vi "Parse SSH_FXP_NAME.vi"(8 "error in":errorcluster, 11 "payload":u8[](array[numeric])) -> (0 "error out":errorcluster, 3 "files":T1[](array[typedef]) {"file attributes"."permissions" format="%04o"})   [LabVIEW 2020, in "NI_SFTP.lvlib"]
uses:
  <vilib>/net/SFTP/NI_SFTP.lvlib
  <vilib>/net/SFTP/API/Support/Name.ctl
  <vilib>/net/SFTP/API/Support/File Attributes.ctl
  f023bfa8-f8fb-3feb-c0fc-b0554016e43f.vi
  fe9cab8e-2cf0-3fe7-1c9b-f8983c6ade3f.vi
  248d59e0-ee9f-3fd5-30f8-f80d1baee43f.vi
  <vilib>/Bit Manipulation/Network-Order Bytes To Words Poly.vi
  <vilib>/Bit Manipulation/wrappers/Network-Order Bytes To Words/Network-Order Bytes To Words U32.vi
  <vilib>/net/SFTP/Low Level Connection/Low Level Connection.lvclass
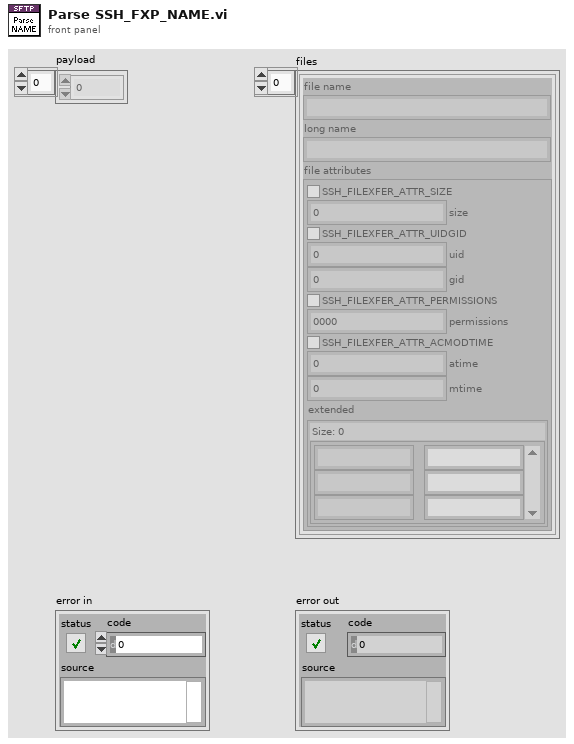
[diagram p1: front panel]
types:
  T1 = typedef "NI_SFTP.lvlib/Name.ctl" = cluster{"file name":string, "long name":string, "file attributes":T2}
  T2 = typedef "NI_SFTP.lvlib/File Attributes.ctl" = cluster{"SSH_FILEXFER_ATTR_SIZE":bool, "size":u64, "SSH_FILEXFER_ATTR_UIDGID":bool, "uid":u32, "gid":u32, "SSH_FILEXFER_ATTR_PERMISSIONS":bool, "permissions":u32, "SSH_FILEXFER_ATTR_ACMODTIME":bool, "atime":u32, "mtime":u32, "extended":map{string, string}}
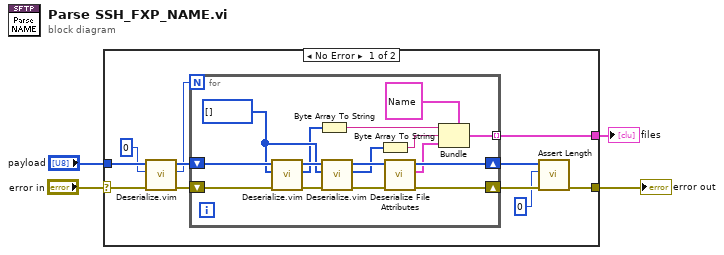
[diagram p0: block diagram]
diagram:
  n1 = case shown="No Error" "error in" {
    selector: "error in" -> [w14 w32]
    tunnel: [w8 w32] -> w3
    tunnel: "payload" -> [w15 _]
    tunnel: [w5 _] -> w1
    frame No Error {
      n2 = call "Deserialize.vim"("error in"=w14, "type"=u32 0, "bytes"=w15) -> ("error out"=w12:errorcluster, "value"=w6:u32, "remaining bytes"=w13:u8[])  [unwired: 6 in]
      n3 = for {
        N: w6 -> [_]
        shift-right: [w24] -> w9
        shift-left: w12 -> [w30]
        shift-right: [w25] -> w10
        shift-left: w13 -> [w31]
        tunnel: [w22] -> w5 mode=indexing
        w20 = u8[] [] ("payload")
        n4 = call "Deserialize.vim"("error in"=w30, "type"=w20, "bytes"=w31) -> ("error out"=w28:errorcluster, "value"=w19:u8[], "remaining bytes"=w29:u8[])  [unwired: 6 in]
        n5 = Byte Array To String(unsigned byte array=w19) -> (string=w18:string)
        n6 = call "Deserialize.vim"("error in"=w28, "type"=w20, "bytes"=w29) -> ("error out"=w26:errorcluster, "value"=w17:u8[], "remaining bytes"=w27:u8[])  [unwired: 6 in]
        n7 = Byte Array To String(unsigned byte array=w17) -> (string=w16:string)
        n8 = call <vilib>:"Deserialize File Attributes.vi"("error in"=w26, "packet"=w27) -> ("error out"=w24:errorcluster, "file attributes"=w23:T2, "packet remaining"=w25:u8[])  [unwired: 7 in]
        n9 = Bundle(cluster=T1 {"file name"="", "long name"="", "file attributes"={"SSH_FILEXFER_ATTR_SIZE"=FALSE, "size"=0, "SSH_FILEXFER_ATTR_UIDGID"=FALSE, "uid"=0, "gid"=0, "SSH_FILEXFER_ATTR_PERMISSIONS"=FALSE, "permissions"=0, "SSH_FILEXFER_ATTR_ACMODTIME"=FALSE, "atime"=0, "mtime"=0, "extended"={}}}, "file name"=w18, "long name"=w16, "file attributes"=w23) -> (w22:T1)
      }
      n10 = call <vilib>:"Assert Length.vi"("error in"=w9, "asserted length"=u32 0, "string in"=w10) -> ("error out"=w8:errorcluster)  [unwired: 7 in, 1 out]
    }
    frame Error {
    }
  }
  "error out" <- w3
  "files" <- w1
